vi "Update Meta data.vi"(8 "error in (no error)":errorcluster, 10 "Meta data":T1[](array[typedef]), 11 "TCP Connection in":refnum<class "TCP Connection.lvclass">) -> (0 "error out":errorcluster, 3 "TCP Connection out":refnum<class "TCP Connection.lvclass">)   [LabVIEW 2018, in "TCP Classes.lvlib" / "TCP Connection.lvclass"]
uses:
  TCP Connection.lvclass
  <vilib>/NI/STM/compatibility/stm_MetaDataElement.ctl
  TCP Connection.lvclass/TCP Connection.ctl
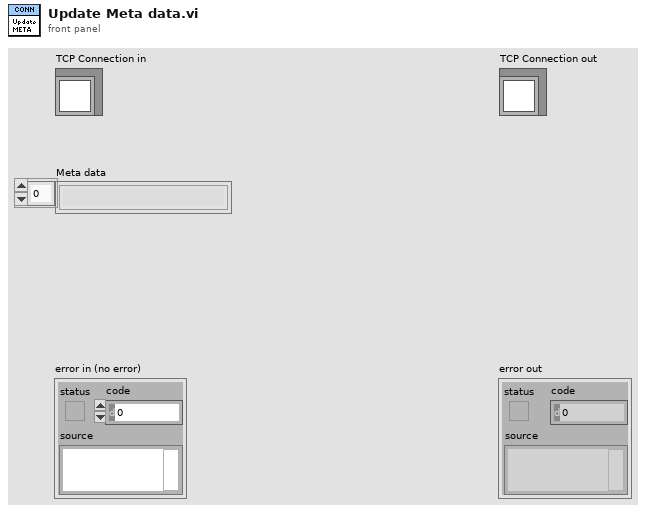
[diagram p1: front panel]
types:
  T1 = typedef "stm_MetaDataElement.ctl" = string
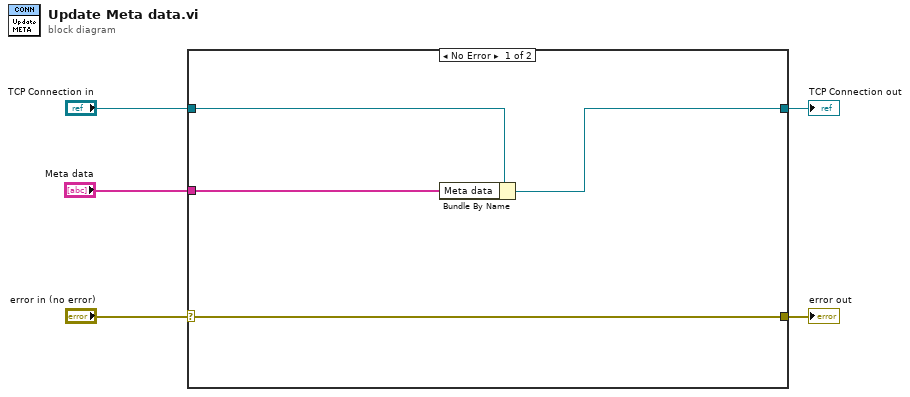
[diagram p0: block diagram]
diagram:
  n1 = case shown="No Error" "error in (no error)" {
    selector: "error in (no error)" -> [w9 w11]
    tunnel: [w9 w11] -> w4
    tunnel: [w7 w10] -> w2
    tunnel: "TCP Connection in" -> [w8 w10]
    tunnel: "Meta data" -> [w6 _]
    frame No Error {
      n2 = Bundle By Name(cluster=w8, "Meta data"=w6) -> (w7:refnum<class "TCP Connection.lvclass">)
    }
    frame Error {
    }
  }
  "error out" <- w4
  "TCP Connection out" <- w2
